vi "Set VI Icon Colour.vi"(6 "VI Path":path, 7 "Type":T1, 8 "error in (no error)":errorcluster) -> (0 "error out":errorcluster)   [LabVIEW 2016]
doc: "Changes the background colour of the vi icon to match the colour requested (plan is to make this match the data type of the assert vi)"
uses:
  <vilib>/Utility/Data Type/Type Definitions/Data Type.ctl
  Icon Colours.ctl
  <vilib>/Utility/Data Type/NI_Data Type.lvlib
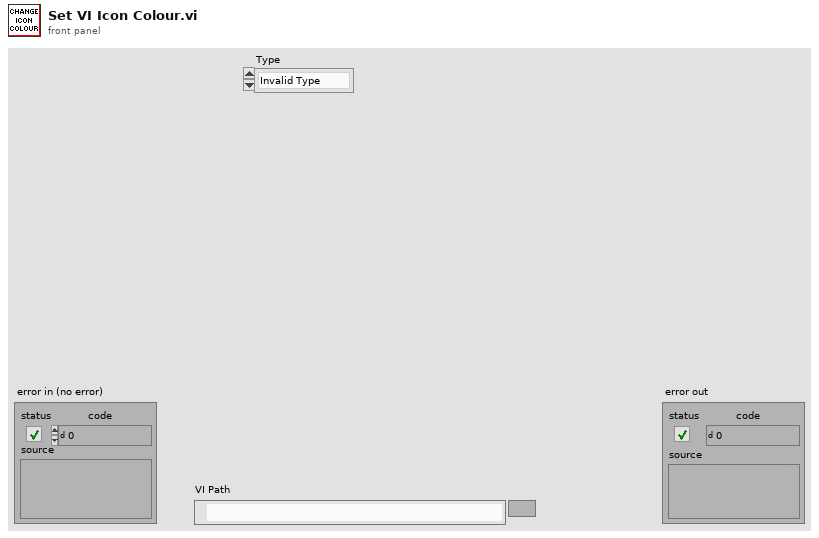
[diagram p1: front panel]
types:
  T1 = typedef "NI_Data Type.lvlib/Data Type.ctl" = enum8{"Invalid Type", "Void", "I8", "I16", "I32", "I64", "U8", "U16", "U32", "U64", "Single Float", "Double Float", "Extended Float", "Single Complex", "Double Complex", "Extended Complex", "Enum U8", "Enum U16", "Enum U32", "Enum U64", "Single Float With Unit", "Double Float With Unit", "Extended Float With Unit", "Single Complex with Unit", "Double Complex with Unit", "Extended Complex with Unit", "Boolean", "String", "Path", "Picture", "Tag", "Array", "Cluster", "Variant", "LV Variant", "Waveform", "Timestamp", "Digital Waveform", "Digital Data", "ExpressData", "Refnum", "External Data", "VI", "Poly VI", "LabVIEW Class Instance", "Fixed Point"}
  T2 = typedef "imagedata.ctl" = cluster{"image type":i32, "image depth":i32, "image":u8[], "mask":u8[], "colors":u32[], "Rectangle":cluster{"left":i16, "top":i16, "right":i16, "bottom":i16}}
  T3 = typedef "Icon Colours.ctl" = string
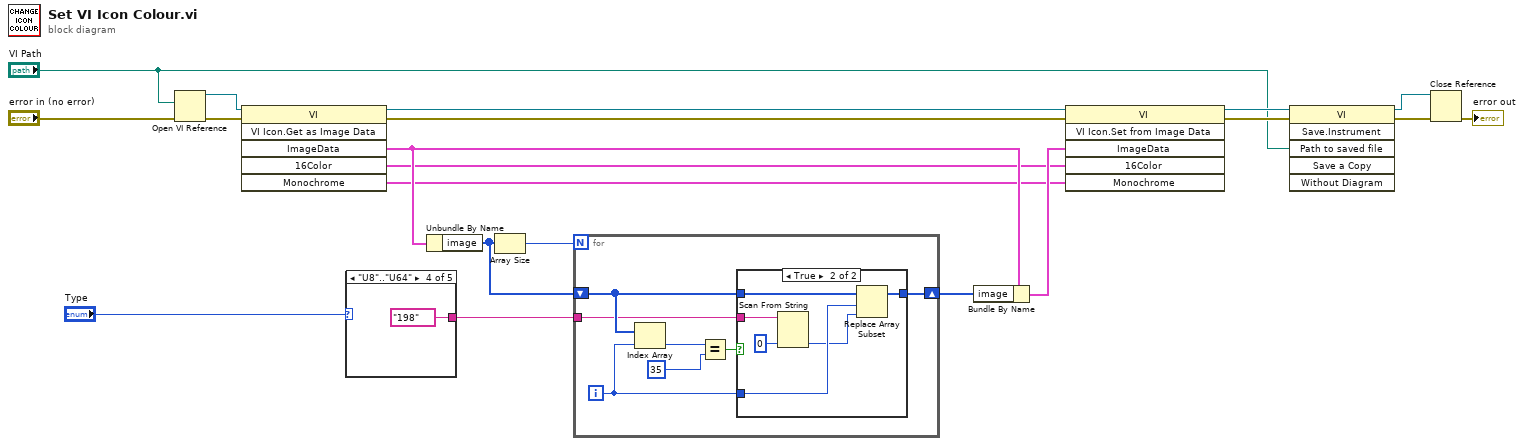
[diagram p0: block diagram]
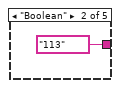
[diagram p3: hidden frame]
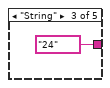
[diagram p4: hidden frame]
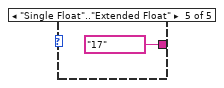
[diagram p5: hidden frame]
diagram:
  n1 = Open VI Reference(vi path="VI Path", error in (no error)="error in (no error)") -> (vi reference=w20:refnum<vi>, error out=w17:errorcluster)  [unwired: 4 in]
  n2 = invoke class="VI" method="VI Icon.Get as Image Data"(reference=w20, error in=w17) -> (reference out=w19:refnum<vi>, error out=w18:errorcluster, "ImageData"=w15:T2, "16Color"=w12:T2, "Monochrome"=w11:T2)  [unwired: 4 in, 1 out]
  n3 = case shown="\"U8\"..\"U64\"" "Type" {
    tunnel: [_ T3 "113" ("Requested Colour") T3 "24" ("Requested Colour") T3 "198" ("Requested Colour") T3 "17" ("Requested Colour")] -> w1
    frame Default {
    }
    frame "Boolean" {
    }
    frame "String" {
    }
    frame "U8".."U64" {
    }
    frame "Single Float".."Extended Float" {
    }
  }
  n4 = Unbundle By Name(w15) -> ("image"=w4:u8[])
  n5 = Array Size(array=w4) -> (size(s)=w3:i32)
  n6 = for {
    N: w3 -> [_]
    shift-right: [w27] -> w14
    shift-left: w4 -> [w29]
    tunnel: w1 -> [w25]
    i -> [w28]
    n7 = Index Array(array=w29, index=w28) -> (element=w30:u8)
    n8 = Equal?(x=w30, y=u8 35) -> (x = y?=w26:bool)
    n9 = case shown="True" w26 {
      tunnel: w29 -> [w32 w38]
      tunnel: w28 -> [_ w36]
      tunnel: [w32 w37] -> w27
      tunnel: w25 -> [_ w35]
      frame False {
      }
      frame True {
        n10 = Scan From String(input string=w35, default 1=u8 0 ("y")) -> (output 1=w33:u8)  [unwired: 3 in, 3 out]
        n11 = Replace Array Subset(array=w38, new element=w33, index=w36) -> (w37:u8[])
      }
    }
  }
  n12 = Bundle By Name(cluster=w15, "image"=w14) -> (w13:T2)
  n13 = invoke class="VI" method="VI Icon.Set from Image Data"(reference=w19, error in=w18, "ImageData"=w13, "16Color"=w12, "Monochrome"=w11) -> (reference out=w10:refnum<vi>, error out=w9:errorcluster)  [unwired: 1 in, 4 out]
  n14 = invoke class="VI" method="Save.Instrument"(reference=w10, error in=w9, "Path to saved file"="VI Path") -> (reference out=w7:refnum<vi>, error out=w6:errorcluster)  [unwired: 3 in, 4 out]
  n15 = Close Reference(reference=w7, error in (no error)=w6) -> (error out=→"error out":errorcluster)
